vi "Untitled 1.vi"() -> ()   [LabVIEW 2018]
panel:
  out "Array 3":bool[](array[boolean])
  in  "Array 5":bool[](array[boolean])
  out "Array 2":dbl[](array[numeric])
  in  "Array":dbl[](array[numeric])
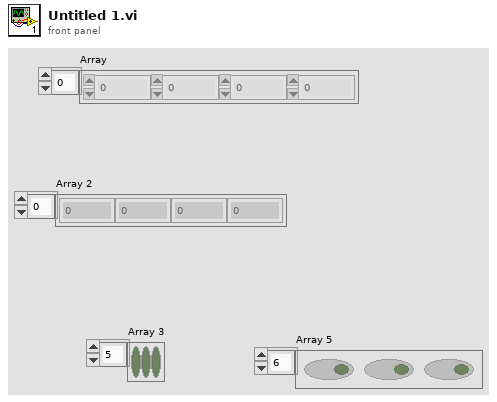
[diagram p1: front panel]
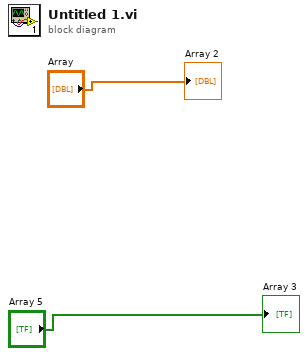
[diagram p0: block diagram]
diagram:
  "Array 2" <- "Array"
  "Array 3" <- "Array 5"
